vi "KernelPCA.vi"(8 "error in":errorcluster) -> (0 "error out":errorcluster, 3 "out":refnum<class "KernelPCA.lvclass">)   [LabVIEW 2020]
doc: "Kernel Principal component analysis (KPCA).\n\n Non-linear dimensionality reduction through the use of kernels (see\n :ref:`metrics`).\n\n Read more in the :ref:`User Guide <kernel_PCA>`.\n\n Parameters\n ----------\n n_components : int, default=None\n Number of components. If None, all non-zero components are kept.\n\n kernel : {'linear', 'poly', 'rbf', 'sigmoid', 'cosine', 'precomputed'}, default='linear'\n Kernel used for PCA.\n\n gamma : float, default=None\n Kernel coefficient for rbf, poly and sigmoid kernels. Ignored by other\n kernels. If ``gamma`` is ``None``, then it is set to ``1/n_features``.\n\n degree : int, default=3\n Degree for poly kernels. Ignored by other kernels.\n\n coef0 : float, default=1\n Independent term in poly and sigmoid kernels.\n Ignored by other kernels.\n\n kernel_params : dict, default=None\n Parameters (keyword arguments) and\n values for kernel passed as callable object.\n Ignored by other kernels.\n\n alpha : float, default=1.0\n Hyperparameter of the ridge regression that learns the\n inverse transform (when fit_inverse_transform=True).\n\n fit_inverse_transform : bool, default=False\n Learn the inverse transform for non-precomputed kernels.\n (i.e. learn to find the pre-image of a point)\n\n eigen_solver : {'auto', 'dense', 'arpack'}, default='auto'\n Select eigensolver to use. If n_components is much less than\n the number of training samples, arpack may be more efficient\n than the dense eigensolver.\n\n tol : float, default=0\n Convergence tolerance for arpack.\n If 0, optimal value will be chosen by arpack.\n\n max_iter : int, default=None\n Maximum number of iterations for arpack.\n If None, optimal value will be chosen by arpack.\n\n remove_zero_eig : bool, default=False\n If True, then all components with zero eigenvalues are removed, so\n that the number of components in the output may be < n_components\n (and sometimes even zero due to numerical instability).\n When n_components is None, this parameter is ignored and components\n with zero eigenvalues are removed regardless.\n\n random_state : int, RandomState instance or None, default=None\n Used when ``eigen_solver`` == 'arpack'. Pass an int for reproducible\n results across multiple function calls.\n See :term:`Glossary <random_state>`.\n\n .. versionadded:: 0.18\n\n copy_X : bool, default=True\n If True, input X is copied and stored by the model in the `X_fit_`\n attribute. If no further changes will be done to X, setting\n `copy_X=False` saves memory by storing a reference.\n\n .. versionadded:: 0.18\n\n n_jobs : int, default=None\n The number of parallel jobs to run.\n ``None`` means 1 unless in a :obj:`joblib.parallel_backend` context.\n ``-1`` means using all processors. See :term:`Glossary <n_jobs>`\n for more details.\n\n .. versionadded:: 0.18\n\n Attributes\n ----------\n lambdas_ : ndarray of shape (n_components,)\n Eigenvalues of the centered kernel matrix in decreasing order.\n If `n_components` and `remove_zero_eig` are not set,\n then all values are stored.\n\n alphas_ : ndarray of shape (n_samples, n_components)\n Eigenvectors of the centered kernel matrix. If `n_components` and\n `remove_zero_eig` are not set, then all components are stored.\n\n dual_coef_ : ndarray of shape (n_samples, n_features)\n Inverse transform matrix. Only available when\n ``fit_inverse_transform`` is True.\n\n X_transformed_fit_ : ndarray of shape (n_samples, n_components)\n Projection of the fitted data on the kernel principal components.\n Only available when ``fit_inverse_transform`` is True.\n\n X_fit_ : ndarray of shape (n_samples, n_features)\n The data used to fit the model. If `copy_X=False`, then `X_fit_` is\n a reference. This attribute is used for the calls to transform.\n\n \nAvailable methods:\nFit\nFit Transform\nTransform\nGet Attributes\nGet Params\nSet Params"
uses:
  KernelPCA.lvclass
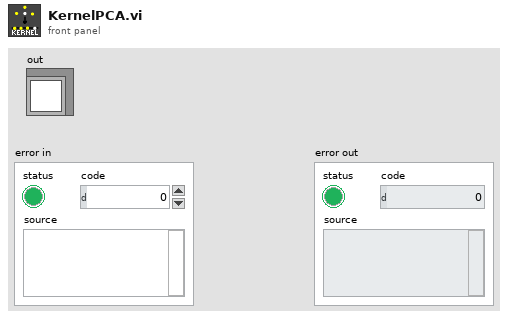
[diagram p1: front panel]
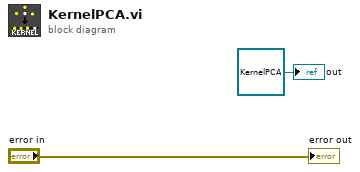
[diagram p0: block diagram]
diagram:
  "out" <- refnum<class "KernelPCA.lvclass"> refnum ("model")
  "error out" <- "error in"
